vi "InitSubSystem.vi"(6 "InitFlags":T1 items=["NONE"=0, "SDL_INIT_AUDIO"=16, "SDL_INIT_VIDEO"=32, "SDL_INIT_JOYSTICK"=512, "SDL_INIT_HAPTIC"=4096, "SDL_INIT_GAMEPAD"=8192, "SDL_INIT_EVENTS"=16384, "SDL_INIT_SENSOR"=32768, "SDL_INIT_CAMER"=65536], 8 "No Error":errorcluster) -> (0 "error out":errorcluster)   [LabVIEW 2024, in "SDL3.lvlib" / "Init.lvlib"]
doc: "<B>Summary</B>\nCompatibility function to initialize the SDL library.\n\n<B>Remarks</B>\nThis function and SDL_Init() are interchangeable."
uses:
  Init.lvlib
  InitFlags--ring.ctl
  Lib/SDL3-32.dll
  Error/Error.lvlib
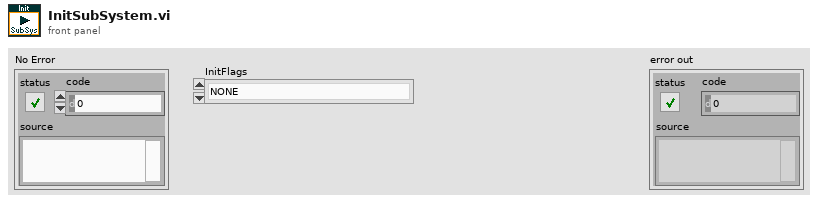
[diagram p1: front panel]
types:
  T1 = typedef "SDL3.lvlib/Init.lvlib/InitFlags--ring.ctl" = u32
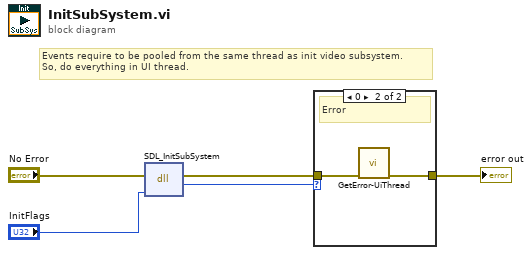
[diagram p0: block diagram]
diagram:
  # "Events require to be pooled from the same thread as init video subsystem.\nSo, do everything in UI thread."
  n1 = dll-call lib="C:/Users/Thomas/Documents/Projects/LV-SDL3/Lib/SDL3-*.*" fn="SDL_InitSubSystem"(error in="No Error", "flags"="InitFlags") -> (error out=w1:errorcluster, "return type"=w2:i32)  [unwired: 3 in, 1 out]
  n2 = case shown="0" w2 {
    tunnel: w1 -> [w6 w8]
    tunnel: [w6 w7] -> w4
    frame Default {
      # "Ok"
    }
    frame 0 {
      # "Error"
      n3 = call "GetError-UiThread.vi"("No Error"=w8) -> ("error out"=w7:errorcluster)  [unwired: 10 in]
    }
  }
  "error out" <- w4
